vi "Open Diagram.vi"(8 "error in (no error)":errorcluster, 10 "DQMH_ARG":T1) -> (0 "error out":errorcluster)   [LabVIEW 2019, in "Peek Window.lvlib"]
doc: "_____\nCreated using Delacor QMH Event Scripter 5.0.0.112."
uses:
  Peek Window.lvlib
  Open Diagram Argument--cluster.ctl
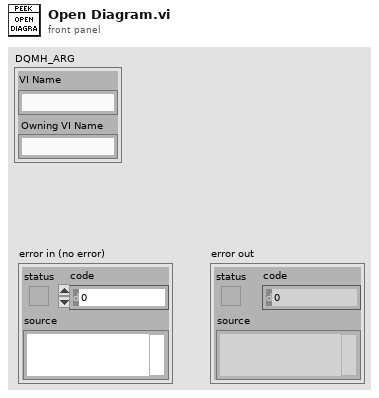
[diagram p1: front panel]
types:
  T1 = typedef "Peek Window.lvlib/Open Diagram Argument--cluster.ctl" = cluster{"VI Name":string, "Owning VI Name":string}
  T2 = typedef "Peek Window.lvlib/Request Events--cluster.ctl" = cluster{"Stop Module":refnum<user-event>, "Show Panel":refnum<user-event>, "Hide Panel":refnum<user-event>, "Get Module Execution Status":refnum<user-event>, "Show Diagram":refnum<user-event>, "Open Diagram":refnum<user-event>}
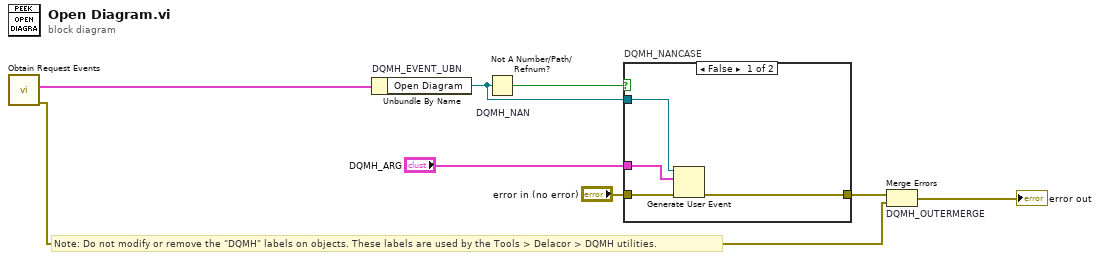
[diagram p0: block diagram]
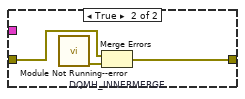
[diagram p2: hidden frame]
diagram:
  # "Note: Do not modify or remove the \"DQMH\" labels on objects. These labels are used by the Tools > Delacor > DQMH utilities."
  n1 = call "Obtain Request Events.vi"() -> ("error out"=w3:errorcluster, "Peek Window Request Events"=w2:T2)  [unwired: 10 in]
  n2 = Unbundle By Name "DQMH_EVENT_UBN"(w2) -> ("Open Diagram"=w5:refnum<user-event>)
  n3 = Not A Number/Path/Refnum? "DQMH_NAN"(number/path/refnum=w5) -> (NaN/Path/Refnum?=w6:bool)
  n4 = case "DQMH_NANCASE" shown="False" w6 {
    tunnel: "error in (no error)" -> [w12 w15]
    tunnel: [w11 w14] -> w4
    tunnel: w5 -> [w10 _]
    tunnel: "DQMH_ARG" -> [w9 _]
    frame False {
      n5 = Generate User Event(user event=w10, event data cluster=w9, error in=w12) -> (error out=w11:errorcluster)  [unwired: 1 in, 1 out]
    }
    frame True {
      n6 = call "Module Not Running--error.vi"() -> ("error out"=w13:errorcluster)  [unwired: 11 in]
      n7 = Merge Errors "DQMH_INNERMERGE"(w15, w13) -> (w14:errorcluster)
    }
  }
  n8 = Merge Errors "DQMH_OUTERMERGE"(w4, w3) -> (→"error out":errorcluster)
